vi "onStart.vi"(8 "error in (no error)":errorcluster, 11 "MeasuringDevice":refnum<class "MeasuringDevice.lvclass">) -> (0 "error out":errorcluster, 3 "MeasuringDevice out":refnum<class "MeasuringDevice.lvclass">)   [LabVIEW 2017, in "MeasuringDevice.lvclass"]
doc: "JKI State Machine Objects (SMO) 1.3.0.56\nJKI - JKI\nCopyright (c) 2017, JKI"
uses:
  MeasuringDevice.lvclass
  <vilib>/JKI/JKI SMO/SMO/SMO.lvclass
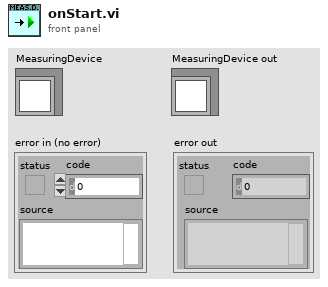
[diagram p1: front panel]
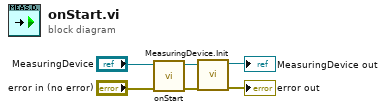
[diagram p0: block diagram]
diagram:
  n1 = call-parent "onStart.vi"("error in (no error)"="error in (no error)", "SMO"="MeasuringDevice") -> ("error out"=w2:errorcluster, "SMO out"=w4:refnum<class "MeasuringDevice.lvclass">)  [unwired: 8 in]
  n2 = call-dynamic "MeasuringDevice.Init.vi"("error in (no error)"=w2, "MeasuringDevice"=w4) -> ("error out"=→"error out":errorcluster, "MeasuringDevice out"=→"MeasuringDevice out":refnum<class "MeasuringDevice.lvclass">)  [unwired: 8 in]
